vi "ReconnectMessage.vi"(8 "error in":errorcluster) -> (0 "error out":errorcluster, 2 "Cancelled":bool)   [LabVIEW 2011]
panel:
  in  "Cancel":bool
  in  "Retry":bool
  # "Could not find any CompactDAQ device!\n\nPlease connect your CompactDAQ device to your computer and Retry..."
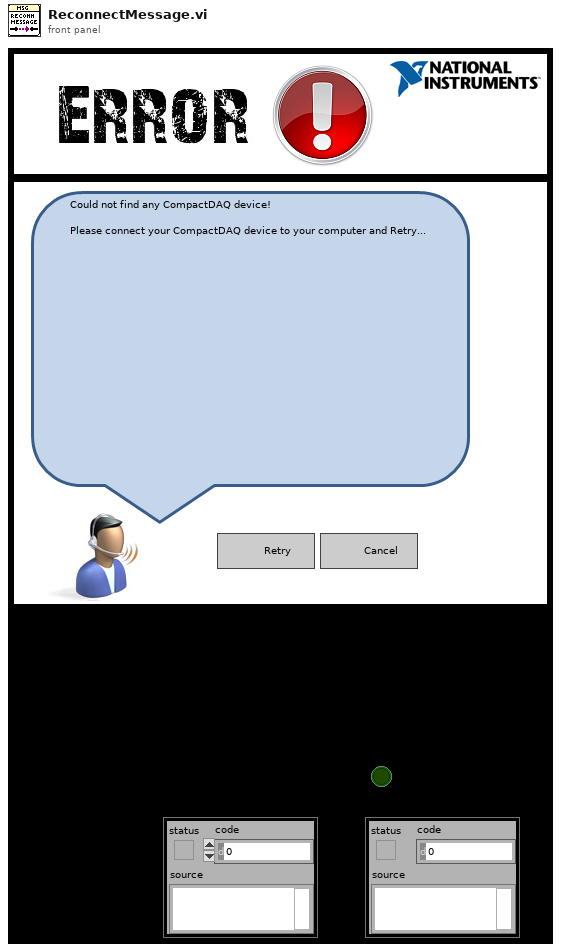
[diagram p1: front panel]
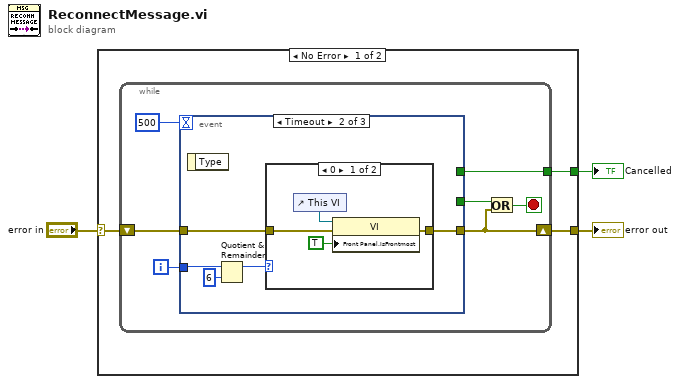
[diagram p0: block diagram]
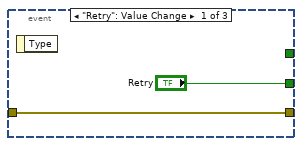
[diagram p2: hidden frame]
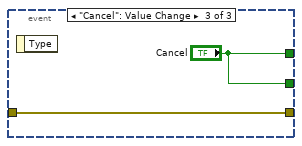
[diagram p4: hidden frame]
diagram:
  n1 = case shown="No Error" "error in" {
    selector: "error in" -> [w4 w28]
    tunnel: [w6 _] -> w3
    tunnel: [w5 w28] -> w2
    frame No Error {
      n2 = while {
        shift-right: [w12] -> w5
        shift-left: w4 -> [w13]
        tunnel: [w9] -> w6
        i -> [w7]
        stop <- w11 stop-if-true
        n3 = event shown="[1] Timeout" {
          selector: _ -> [_ _ _]
          dyn-events: _ -> [_ _ _]
          timeout: 500 -> [_ _ _]
          tunnel: w13 -> [w14 w20 w26]
          tunnel: [w14 w19 w26] -> w12
          tunnel: ["Retry" _ "Cancel"] -> w10
          tunnel: [_ _ "Cancel"] -> w9
          tunnel: w7 -> [_ w18 _]
          event "Retry": Value Change {
            n4 = event-data() -> ()  [unwired: 1 in, 1 out]
          }
          event Timeout {
            n5 = event-data() -> ()  [unwired: 1 in, 1 out]
            n6 = Quotient & Remainder(x=w18, y=6) -> (x-y*floor(x/y)=w16:i32)  [unwired: 1 out]
            n7 = case shown="0" w16 {
              tunnel: w20 -> [w23 w25]
              tunnel: [w24 w25] -> w19
              frame 0 {
                n8 = control-ref of="This VI"() -> (w22:refnum<vi>)
                n9 = property class="VI"(reference=w22, error in=w23, "Front Panel.IsFrontmost"=TRUE ("Front Panel Window:Is Frontmost")) -> (error out=w24:errorcluster)  [unwired: 1 out]
              }
              frame Default {
              }
            }
          }
          event "Cancel": Value Change {
            n10 = event-data() -> ()  [unwired: 1 in, 1 out]
          }
        }
        n11 = Or(x=w10, y=w12) -> (x .or. y?=w11:bool)
      }
    }
    frame Error {
    }
  }
  "Cancelled" <- w3
  "error out" <- w2
